vi "Global State Variables.vi"() -> ()   [LabVIEW 2017]
panel:
  out "BiStateVariableSwitched":bool
  in  "BiStateVariable":enum16{"State1", "State2"}(ring)
  in  "DriveSpeedRange":enum16{"DriveSpeedHigh", "DriveSpeedLow"}(ring)
  in  "WinchState":enum16{"WinchOff", "WinchClimb", "WinchHold"}(ring)
  in  "Camera Selected":enum16{"Peg Camera", "Rope Camera"}(ring)
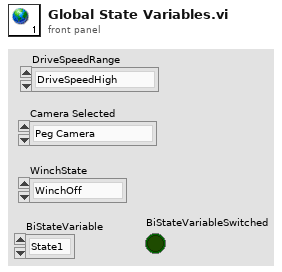
[diagram p1: front panel]
diagram:
